vi "STD二氧化碳分压（pCO2）走航观测系统.vi"() -> ()   [LabVIEW 2016]
panel:
  out "字符串":string
  in  "打开文件":bool
  in  "开始测量":bool
  in  "编辑步骤":bool
  in  "设备配置&联机按钮":bool
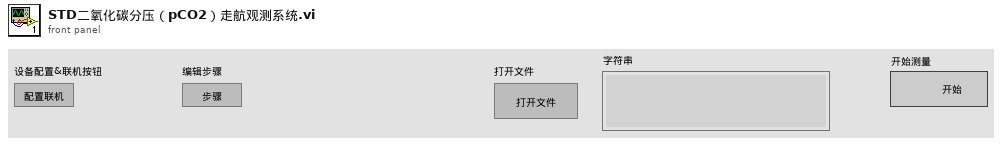
[diagram p1: front panel]
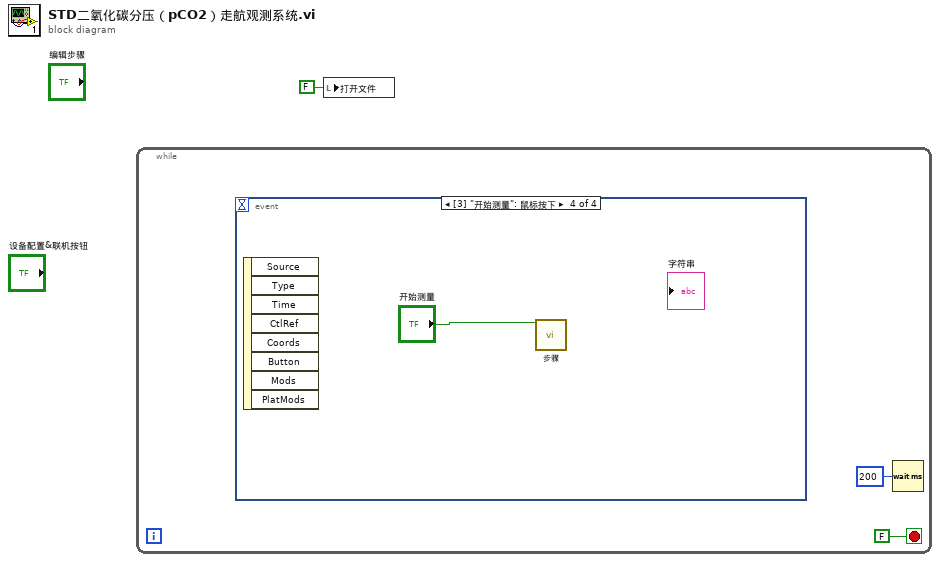
[diagram p0: block diagram]
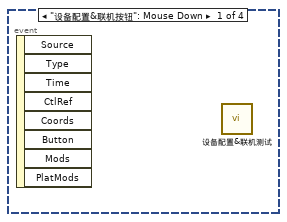
[diagram p2: hidden frame]
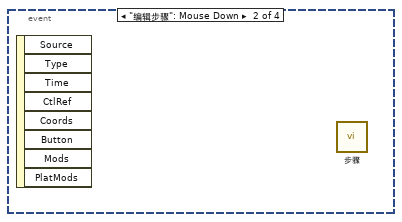
[diagram p3: hidden frame]
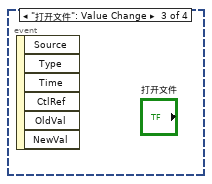
[diagram p4: hidden frame]
diagram:
  n1 = while {
    stop <- FALSE stop-if-true
    n2 = event shown="[3] \"开始测量\": 鼠标按下" {
      selector: _ -> [_ _ _ _]
      dyn-events: _ -> [_ _ _ _]
      timeout: _ -> [_ _ _ _]
      event "设备配置&联机按钮": Mouse Down {
        n3 = event-data() -> ()  [unwired: 1 in, 8 out]
        n4 = call "设备配置&联机测试.vi"() -> ()  [unwired: 11 in, 1 out]
      }
      event "编辑步骤": Mouse Down {
        n5 = event-data() -> ()  [unwired: 1 in, 8 out]
        n6 = call "步骤.vi"() -> ()  [unwired: 11 in, 5 out]
      }
      event "打开文件": Value Change {
        n7 = event-data() -> ()  [unwired: 1 in, 6 out]
      }
      event "开始测量": Mouse Down {
        n8 = event-data() -> ()  [unwired: 1 in, 8 out]
        n9 = call "步骤.vi"("开始"="开始测量") -> ()  [unwired: 10 in, 5 out]
      }
    }
    n10 = Wait (ms)(milliseconds to wait=u32 200 ("等待时间（毫秒）")) -> ()  [unwired: 1 out]
  }
  n11 = local write "打开文件"(FALSE ("打开文件")) -> ()
